vi "initial.vi"(8 "error in (no error)":errorcluster, 11 "DMC1000B in":refnum<class "DMC1000B.lvclass">) -> (0 "error out":errorcluster, 3 "DMC1000B out":refnum<class "DMC1000B.lvclass">)   [LabVIEW 2019, in "DMC1000B.lvclass"]
uses:
  DMC1000B.lvclass
  IOCard.lvclass/IOCard.ctl
  IOCard.lvclass
  LLB/DMC1000B/Dmc1000/Dmc1000.lvlib
  LLB/Commonly VI.lvlib
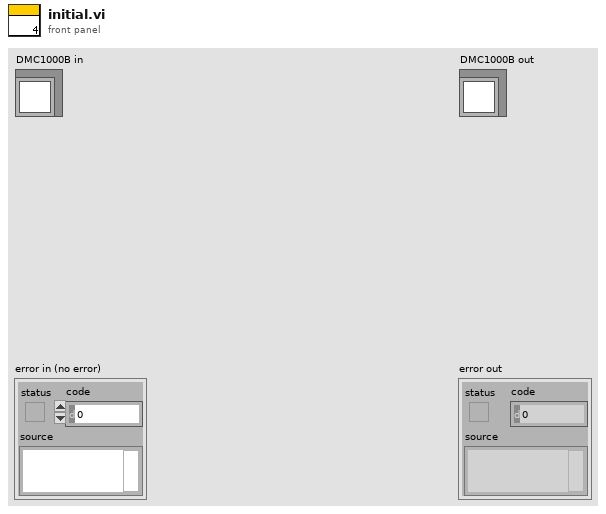
[diagram p1: front panel]
types:
  T1 = typedef "IO Card_Type.ctl" = enum16{"None", "Unidaq32", "6480", "2410C-64", "Zan", "DMC1000B", "16InOut", "Robot", "DMC3600"}
  T2 = cluster{"IO Card Type":T1, "IOType":enum16{"Input", "Output"}, "CardNumber":i32, "ConnectAct":bool, "IP":string}
  T3 = cluster{"CardNumber":i32, "Connect":bool, "Handler":i32}
  T4 = cluster{"Card":i32, "Connect":bool, "Handler":i32}[]
  T5 = cluster{"Card":i32, "Connect":bool, "Handler":i32}
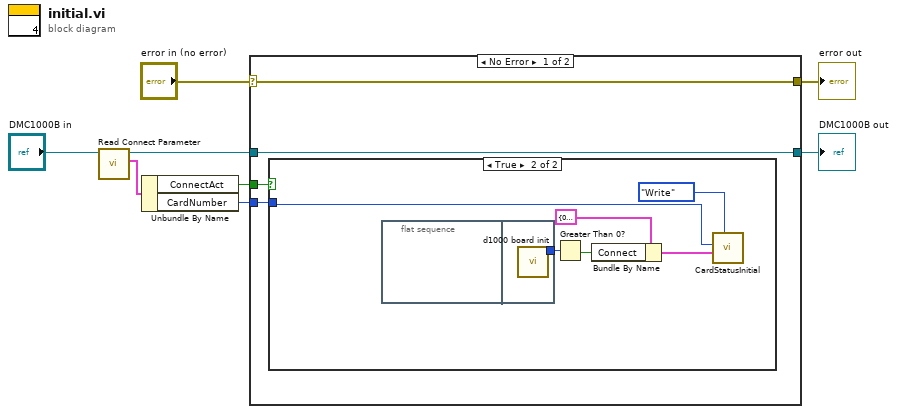
[diagram p0: block diagram]
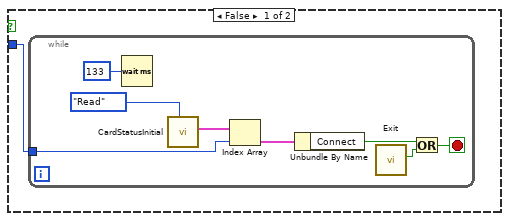
[diagram p2: hidden frame]
diagram:
  n1 = call "Read Connect Parameter.vi"("IOCard in"="DMC1000B in") -> ("Connect Parameter"=w6:T2, "IOCard out"=w4:refnum<class "DMC1000B.lvclass">)  [unwired: 8 in, 1 out]
  n2 = Unbundle By Name(w6) -> ("ConnectAct"=w5:bool, "CardNumber"=w3:i32)
  n3 = case shown="No Error" "error in (no error)" {
    selector: "error in (no error)" -> [w9 w29]
    tunnel: w5 -> [w12 _]
    tunnel: w4 -> [w10 w30]
    tunnel: w3 -> [w11 _]
    tunnel: [w10 w30] -> w2
    tunnel: [w9 w29] -> w1
    frame No Error {
      n4 = case shown="True" w12 {
        tunnel: w11 -> [w13 w24]
        frame False {
          n5 = while {
            tunnel: w13 -> [w19]
            stop <- w15 stop-if-true
            n6 = Wait (ms)(milliseconds to wait=u32 133 ("millisecond timer value")) -> ()  [unwired: 1 out]
            n7 = call "CardStatusInitial.vi"("Action"=enum16{"Initial", "Write", "Read", "Release"}."Read") -> ("CardStatus"=w20:T4)  [unwired: 10 in]
            n8 = Index Array(array=w20, index=w19) -> (element=w18:T5)
            n9 = Unbundle By Name(w18) -> ("Connect"=w17:bool)
            n10 = call "Exit.vi"() -> ("ExitOut"=w16:bool)  [unwired: 11 in]
            n11 = Or(x=w17, y=w16) -> (x .or. y?=w15:bool)
          }
        }
        frame True {
          n12 = flat-sequence {
            tunnel: [w28] -> w27
            frame #0 {
            }
            frame #1 {
              n13 = call "d1000 board init.vi"() -> ("function return"=w28:u32)  [unwired: 11 in]
            }
          }
          n14 = Greater Than 0?(x=w27) -> (x > 0?=w22:bool)
          n15 = Bundle By Name(cluster=T3 {"CardNumber"=0, "Connect"=FALSE, "Handler"=0} ("DataIn"), "Connect"=w22) -> (w23:T3)
          n16 = call "CardStatusInitial.vi"("Action"=enum16{"Initial", "Write", "Read", "Release"}."Write", "DataIn"=w23, "CardNumber"=w24) -> ()  [unwired: 8 in, 1 out]
        }
      }
    }
    frame Error {
    }
  }
  "error out" <- w1
  "DMC1000B out" <- w2
